vi "Periodic Tasks.vi"(8 "error in":errorcluster) -> ()   [LabVIEW 2017]
doc: "This VI runs in parallel to other robot code. It can contain as many user-defined periodic loops as you need. These can carry out PID or other sorts of timed response."
uses:
  <vilib>/Rock Robotics/WPI/Utilities/WPI_GetSetVariantRefNum.vi
  <vilib>/Rock Robotics/WPI/Ultrasonic/WPI_SonarMB1010AnalogRefNum Registry Get.vi
  <vilib>/Rock Robotics/WPI/Ultrasonic/WPI_SonarMB1010AnalogGetRange.vi
  Robot Global Data.vi
  <vilib>/Rock Robotics/WPI/ThirdParty/Sensors/ADIS16448 IMU/ADIS16448_IMU.lvlib
panel:
  out "IMU Angles Out":T1
  out "Z Angle":dbl
  out "Sonar Distance":dbl
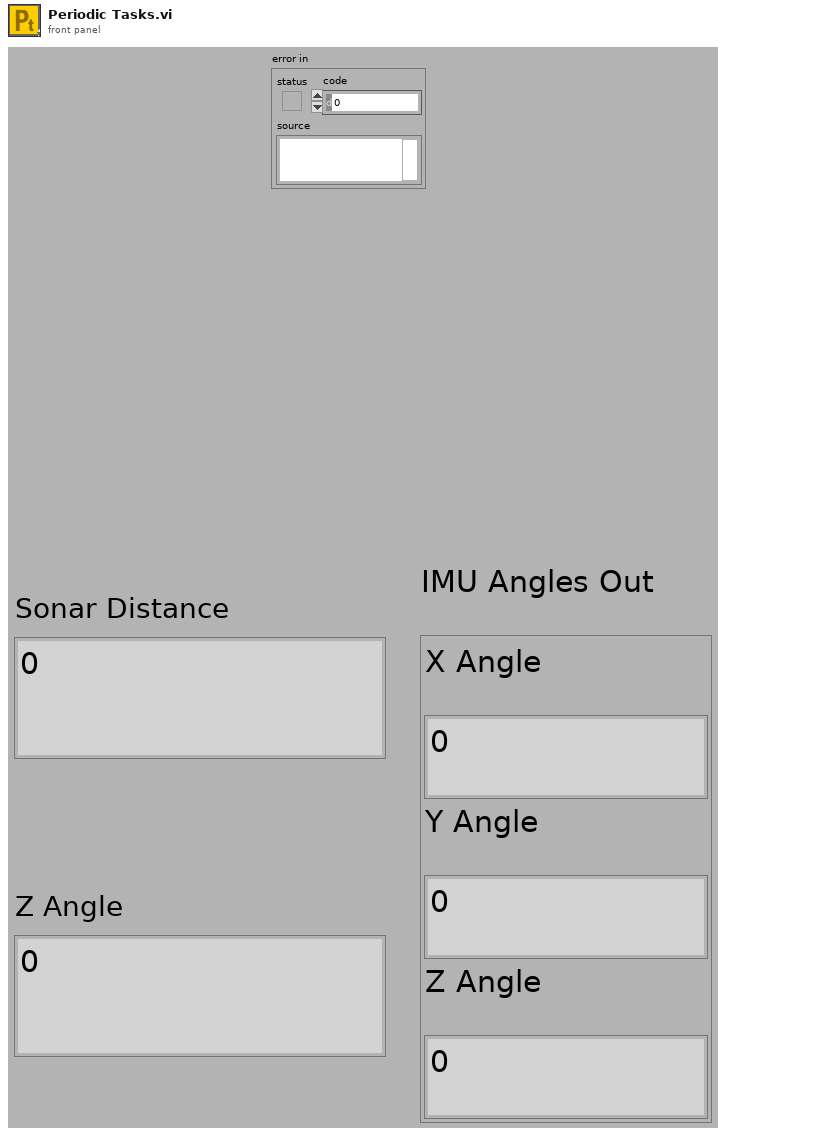
[diagram p1: front panel]
types:
  T1 = cluster{"X Angle":dbl, "Y Angle":dbl, "Z Angle":dbl}
  T2 = typedef "WPI_SonarMB1010AnalogDeviceRef.ctl" = cluster{"AIDeviceRef":T3, "Scaling factor (V/in)":dbl, "Average Bits":u8}
  T3 = typedef "WPI_AnalogChannelDevRef.ctl" = cluster{"DevStatus":errorcluster, "Analog Channel":T4}
  T4 = typedef "FPGA_AIChannel.ctl" = enum8{"AI 0", "AI 1", "AI 2", "AI 3", "AI MXP 0", "AI MXP 1", "AI MXP 2", "AI MXP 3", "Invalid"}
  T5 = typedef "ADIS16448_IMU.lvlib/ADI_IMU_ADIS16448_IMUDevRef.ctl" = cluster{"DevStatus":errorcluster, "Handle":i32, "SPI Bus":T6, "Device Found":bool, "Device Ready":bool, "Yaw Axis":enum16{"X", "Y", "Z"}, "AHRS Algorithm":enum16{"Complementary", "Madgwick"}, "Serial":u16, "Lot ID 2":u16, "Lot ID 1":u16, "Bytes Per Sample":u16, "Calibrate On Open?":bool}
  T6 = typedef "spi_bus.ctl" = enum16{"SPI On-Board, CS0", "SPI On-Board, CS1", "SPI On-Board, CS2", "SPI On-Board, CS3", "SPI MXP", "Invalid"}
  T7 = typedef "WPI_JoystickDevRef.ctl" = cluster{"Device":T8}
  T8 = typedef "WPI_JoystickDeviceEnum.ctl" = enum16{"USB 0", "USB 1", "USB 2", "USB 3", "USB 4", "USB 5"}
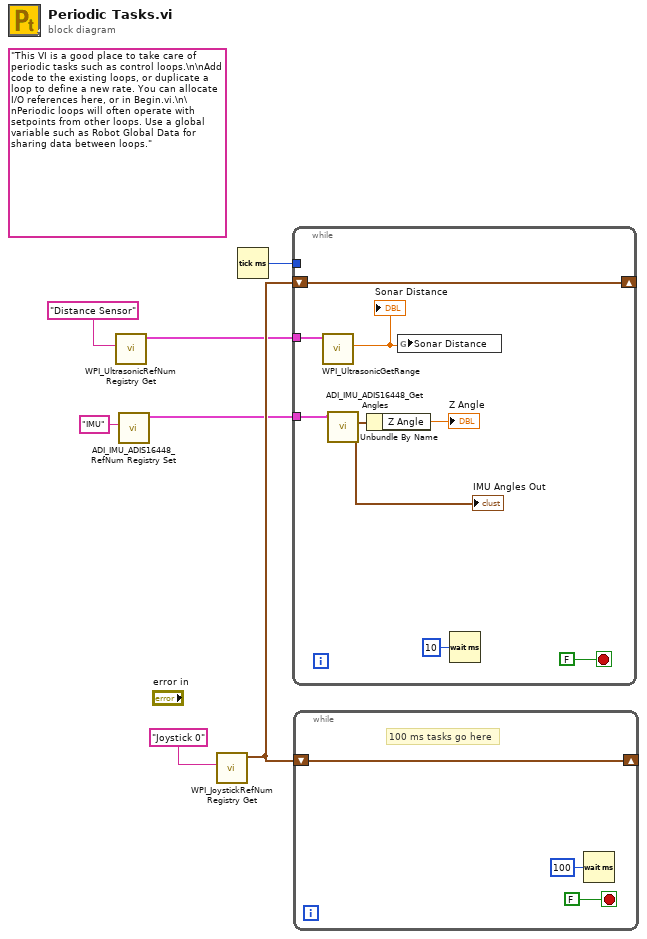
[diagram p0: block diagram]
diagram:
  (unwired) "This VI is a good place to take care of periodic tasks such as control loops.\n\nAdd code to the existing loops, or duplicate a loop to define a new rate. You can allocate I/O references here, or in Begin.vi.\n\nPeriodic loops will often operate with setpoints from other loops. Use a global variable such as Robot Global Data for sharing data between loops."
  n1 = call-poly <vilib>:"WPI_UltrasonicRefNum Registry Get.vi"("refnum name"="Distance Sensor") -> ("SonarMB1010AnalogDevRef"=w3:T2)  [unwired: 9 in, 1 out]
  n2 = call <vilib>:"ADI_IMU_ADIS16448_RefNum Registry Set.vi"("refnum name"="IMU") -> ("ADI IMU DevRef"=w1:T5)  [unwired: 9 in, 1 out]
  n3 = call <vilib>:"WPI_JoystickRefNum Registry Get.vi"("refnum name"="Joystick 0") -> ("JoystickDevRef"=w6:T7)  [unwired: 1 in, 9 out]
  n4 = Tick Count (ms)() -> (millisecond timer value=w5:u32)
  n5 = while {
    shift-right: [w14] -> _
    shift-left: w6 -> [w14]
    tunnel: w5 -> [_]
    tunnel: w3 -> [w12]
    tunnel: w1 -> [w9]
    stop <- FALSE stop-if-true
    n6 = call-poly <vilib>:"WPI_UltrasonicGetRange.vi"("SonarMB1010AnalogDevRef"=w12) -> ("Distance"=w11:dbl)  [unwired: 8 in, 2 out]
    "Sonar Distance" <- w11
    n7 = call <vilib>:"ADI_IMU_ADIS16448_Get Angles.vi"("ADI IMU DevRef"=w9) -> ("IMU Angles Out"=w10:T1)  [unwired: 7 in, 3 out]
    "IMU Angles Out" <- w10
    n8 = Unbundle By Name(w10) -> ("Z Angle"=→"Z Angle":dbl)
    n9 = global write "Robot Global Data.vi" "Sonar Distance"(w11) -> ()
    n10 = Wait (ms)(milliseconds to wait=u32 10) -> ()  [unwired: 1 out]
  }
  n11 = while {
    shift-right: [w16] -> _
    shift-left: w6 -> [w16]
    stop <- FALSE stop-if-true
    # "100 ms tasks go here"
    n12 = Wait (ms)(milliseconds to wait=u32 100) -> ()  [unwired: 1 out]
  }
